vi "Robot Global Data.vi"() -> ()   [LabVIEW 2015]
doc: "This global VI can contain as many global variables as you need. Place a control on the panel, give it a good name. To read or write to it from a VI, drag the icon to the diagram of that VI. You can also drag from the project. Click on the node to change which global you access. You shouldn't have multiple locations writing to a global or it will cause a race-condition."
uses:
  <vilib>/Rock Robotics/WPI/DriverStation/WPI_DriverStationRobotMode2.ctl
panel:
  out "Rio to Dash":cluster{"Recording?":bool, "Running?":bool}
  out "Dash to Rio":T1
  in  "Hold drive":bool
  in  "All":T2
  in  "Robot Mode":T3
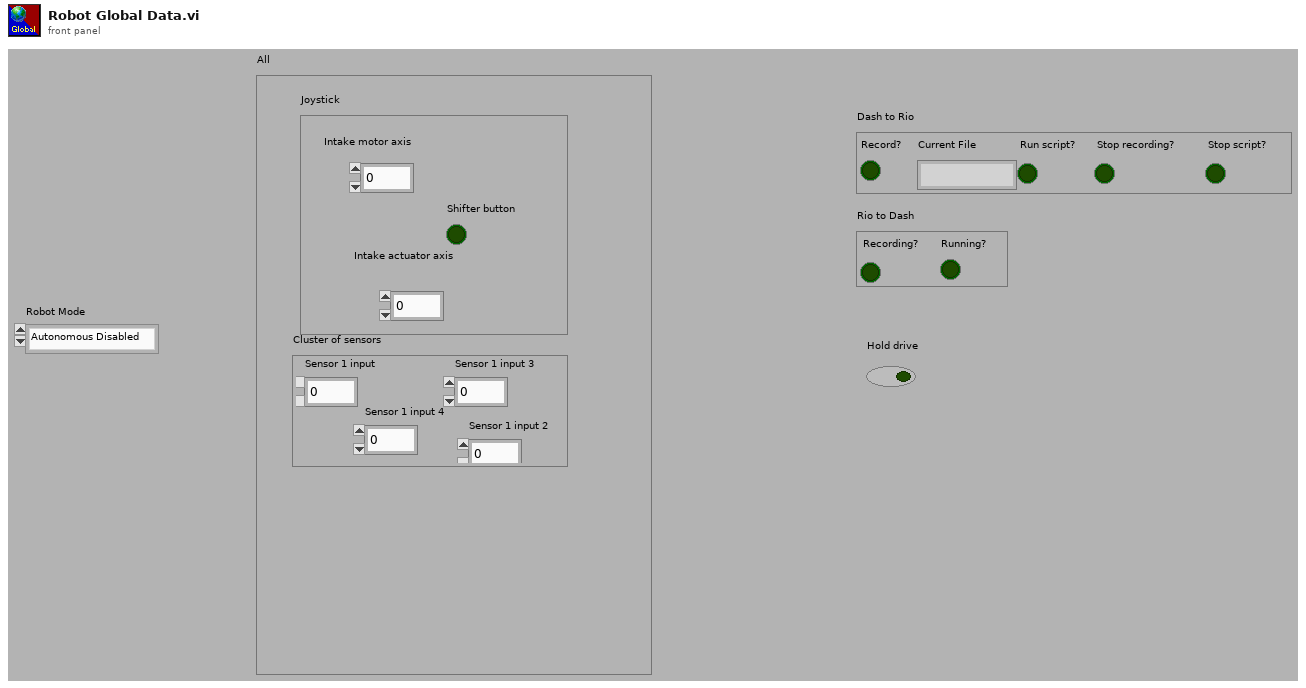
[diagram p1: front panel]
types:
  T1 = cluster{"Record?":bool, "Current File":string, "Run script?":bool, "Stop recording?":bool, "Stop script?":bool}
  T2 = cluster{"Joystick":cluster{"Intake motor axis":dbl, "Intake actuator axis":dbl, "Shifter button":bool}, "Cluster of sensors":cluster{"Sensor 1 input 2":u8, "Sensor 1 input 3":u8, "Sensor 1 input":u8, "Sensor 1 input 4":u8}}
  T3 = typedef "WPI_DriverStationRobotMode2.ctl" = enum16{"Autonomous Disabled", "Autonomous Enabled", "Teleop Disabled", "Teleop Enabled", "Disconnected", "Finish", "Test Disabled", "Test Enabled", "Emergency Stopped"}
diagram:
